vi "Runtime.vi"(11 "Script in 2d":string[][](array[string])) -> (3 "Runtime":dbl)   [LabVIEW 2015]
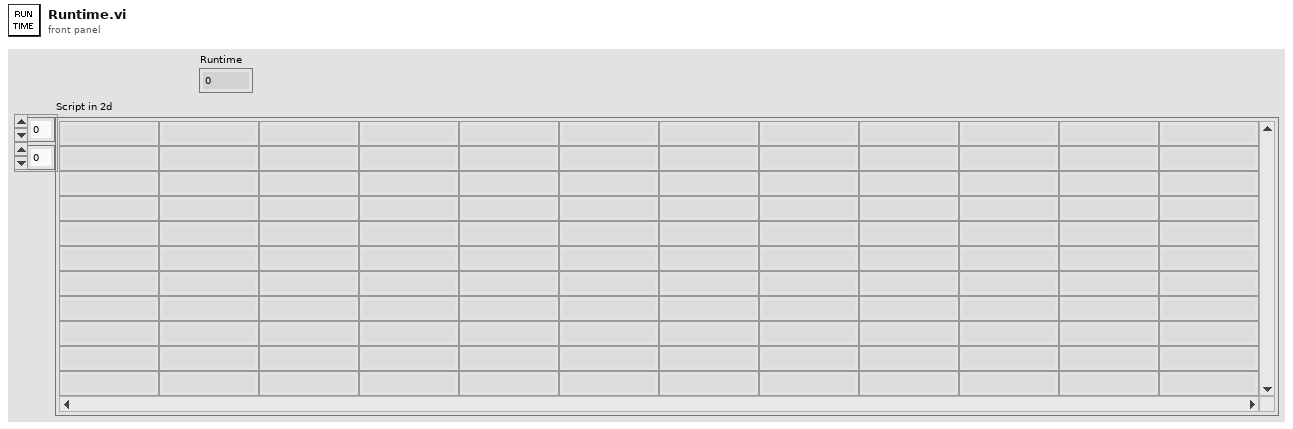
[diagram p1: front panel]
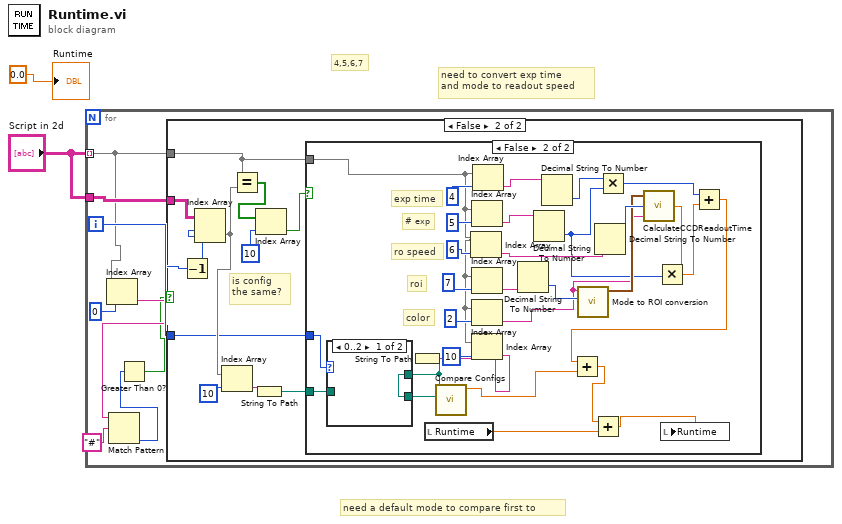
[diagram p0: block diagram]
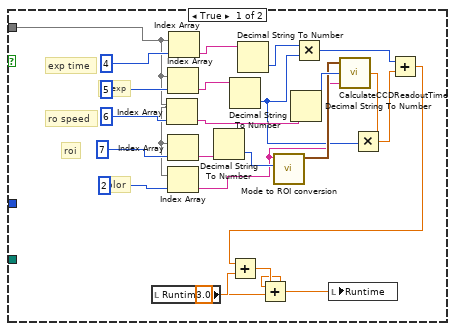
[diagram p3: hidden frame]
diagram:
  # "need a default mode to compare first to"
  # "4,5,6,7"
  # "need to convert exp time\nand mode to readout speed"
  n1 = for {
    tunnel: "Script in 2d" -> [w5] mode=indexing
    tunnel: "Script in 2d" -> [w10]
    i -> [w9]
    n2 = Index Array(array=w5, index=0) -> (element=w4:string)
    n3 = Match Pattern(string=w4, regular expression="#") -> (offset past match=w6:i32)  [unwired: 1 in, 3 out]
    n4 = Greater Than 0?(x=w6) -> (x > 0?=w3:bool)
    n5 = case shown="False" w3 {
      tunnel: w5 -> [_ w21]
      tunnel: w10 -> [_ w20]
      tunnel: w9 -> [_ w11]
      frame True {
        # "skip commented lines"
      }
      frame False {
        # "is config \nthe same?"
        n6 = Decrement(x=w11) -> (x-1=w19:i32)
        n7 = Index Array(array=w20, index (row)=w19) -> (element=w14:string[])  [unwired: 1 in]
        n8 = Index Array(array=w14, index=10) -> (element=w13:string)
        n9 = Equal?(x=w21, y=w14) -> (x = y?=w18:bool[])
        n10 = String To Path(string=w13) -> (path=w12:path)
        n11 = Index Array(array=w18, index=10) -> (element=w16:bool)
        n12 = case shown="False" w16 {
          tunnel: w21 -> [w36 w53]
          tunnel: w12 -> [_ w48]
          tunnel: w11 -> [_ w49]
          frame True {
            # "exp time"
            # "# exp"
            # "ro speed"
            # "roi"
            # "color"
            n13 = local read "Runtime"() -> (w45:dbl)
            n14 = Index Array(array=w36, index=6) -> (element=w34:string)
            n15 = Index Array(array=w36, index=5) -> (element=w29:string)
            n16 = Index Array(array=w36, index=7) -> (element=w33:string)
            n17 = Index Array(array=w36, index=2) -> (element=w30:string)
            n18 = Index Array(array=w36, index=4) -> (element=w28:string)
            n19 = Decimal String To Number(string=w33) -> (number=w32:i32)  [unwired: 2 in, 1 out]
            n20 = Decimal String To Number(string=w29) -> (number=w25:i32)  [unwired: 2 in, 1 out]
            n21 = Decimal String To Number(string=w28) -> (number=w26:i32)  [unwired: 2 in, 1 out]
            n22 = call "Mode to ROI conversion.vi"("Mode"=w32, "Color"=w30) -> ("CCD ROI"=w31:cluster{i32, i32, i32, i32, i32, i32})  [unwired: 9 in]
            n23 = Decimal String To Number(string=w34) -> (number=w41:i32)  [unwired: 2 in, 1 out]
            n24 = Multiply(x=w26, y=w25) -> (x*y=w24:i32)
            n25 = call "CalculateCCDReadoutTime.vi"("Color"=w30, "Readout Speed"=w41, "CCD ROI"=w31) -> ("Readout Time"=w27:dbl)
            n26 = Multiply(x=w27, y=w25) -> (x*y=w23:dbl)
            n27 = Add(x=w24, y=w23) -> (x+y=w22:dbl)
            n28 = Add(x=w22, y=w45) -> (x+y=w44:dbl)
            n29 = Add(x=3.0, y=w44) -> (x+y=w42:dbl)
            n30 = local write "Runtime"(w42) -> ()
          }
          frame False {
            # "exp time"
            # "# exp"
            # "ro speed"
            # "roi"
            # "color"
            n31 = local read "Runtime"() -> (w75:dbl)
            n32 = Index Array(array=w53, index=6) -> (element=w67:string)
            n33 = Index Array(array=w53, index=5) -> (element=w62:string)
            n34 = Index Array(array=w53, index=7) -> (element=w66:string)
            n35 = Index Array(array=w53, index=2) -> (element=w63:string)
            n36 = Index Array(array=w53, index=10) -> (element=w52:string)
            n37 = String To Path(string=w52) -> (path=w46:path)
            n38 = case shown="0..2" w49 {
              tunnel: w48 -> [_ w77]
              tunnel: [w76 w77] -> w47
              tunnel: w46 -> [w76 _]
              frame 0..2 {
              }
              frame 3, Default {
              }
            }
            n39 = call "Compare Configs.vi"("Old Config"=w47, "New Config"=w46) -> ("Time"=w51:dbl)  [unwired: 9 in]
            n40 = Index Array(array=w53, index=4) -> (element=w61:string)
            n41 = Decimal String To Number(string=w66) -> (number=w65:i32)  [unwired: 2 in, 1 out]
            n42 = Decimal String To Number(string=w62) -> (number=w58:i32)  [unwired: 2 in, 1 out]
            n43 = Decimal String To Number(string=w61) -> (number=w59:i32)  [unwired: 2 in, 1 out]
            n44 = call "Mode to ROI conversion.vi"("Mode"=w65, "Color"=w63) -> ("CCD ROI"=w64:cluster{i32, i32, i32, i32, i32, i32})  [unwired: 9 in]
            n45 = Decimal String To Number(string=w67) -> (number=w73:i32)  [unwired: 2 in, 1 out]
            n46 = Multiply(x=w59, y=w58) -> (x*y=w57:i32)
            n47 = call "CalculateCCDReadoutTime.vi"("Color"=w63, "Readout Speed"=w73, "CCD ROI"=w64) -> ("Readout Time"=w60:dbl)
            n48 = Multiply(x=w60, y=w58) -> (x*y=w56:dbl)
            n49 = Add(x=w57, y=w56) -> (x+y=w55:dbl)
            n50 = Add(x=w55, y=w51) -> (x+y=w50:dbl)
            n51 = Add(x=w50, y=w75) -> (x+y=w74:dbl)
            n52 = local write "Runtime"(w74) -> ()
          }
        }
      }
    }
  }
  "Runtime" <- 0.0
